vi "Get PK Info.vi"(8 "error in (no error)":errorcluster, 11 "FK Ring in":refnum<class "FK Ring.lvclass">) -> (0 "error out":errorcluster, 3 "FK Ring out":refnum<class "FK Ring.lvclass">)   [LabVIEW 2020, in "FK Ring.lvclass"]
uses:
  FK Ring.lvclass
  C:/Users/User/Desktop/Raman Program/Database OOP/source/Field/Field.lvclass
  Field/Field.lvclass/Field.ctl
  FK Ring.lvclass/FK Ring.ctl
  Database/Database.lvclass
  Field/Field.lvclass
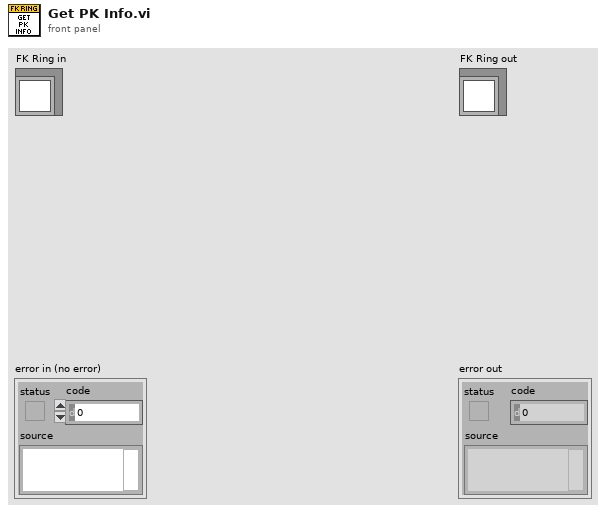
[diagram p1: front panel]
types:
  T1 = typedef "foreign key properties.ctl" = cluster{"FK Table":string, "FK Column":string, "PK Table":string, "PK Column":string, "PK Display Column":string}
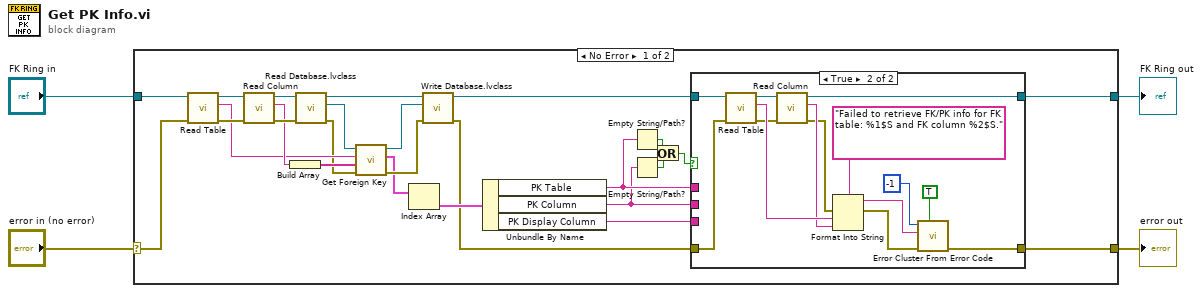
[diagram p0: block diagram]
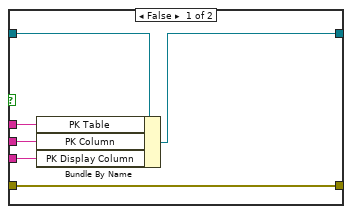
[diagram p2: hidden frame]
diagram:
  n1 = case shown="No Error" "error in (no error)" {
    selector: "error in (no error)" -> [w26 w52]
    tunnel: [w7 w52] -> w3
    tunnel: [w5 w51] -> w1
    tunnel: "FK Ring in" -> [w30 w51]
    frame No Error {
      n2 = call "Read Table.vi"("error in (no error)"=w26, "Field in"=w30) -> ("error out"=w25:errorcluster, "Table"=w22:string, "Field out"=w29:refnum<class "FK Ring.lvclass">)  [unwired: 7 in]
      n3 = call "Read Column.vi"("error in (no error)"=w25, "Field in"=w29) -> ("error out"=w24:errorcluster, "Column"=w23:string, "Field out"=w28:refnum<class "FK Ring.lvclass">)  [unwired: 7 in]
      n4 = Build Array(w23) -> (w21:string[])
      n5 = call "Read Database.lvclass.vi"("error in (no error)"=w24, "Field in"=w28) -> ("error out"=w18:errorcluster, "Database.lvclass"=w20:refnum<class "Database.lvclass">, "Field out"=w27:refnum<class "FK Ring.lvclass">)  [unwired: 7 in]
      n6 = call-dynamic "Get Foreign Key.vi"("error in (no error)"=w18, "Column Name Array"=w21, "Table Name"=w22, "Database in"=w20) -> ("error out"=w17:errorcluster, "FK Properties Array"=w16:T1[], "Database out"=w19:refnum<class "Database.lvclass">)  [unwired: 5 in]
      n7 = Index Array(array=w16) -> (element=w15:T1)  [unwired: 1 in]
      n8 = call "Write Database.lvclass.vi"("error in (no error)"=w17, "Database.lvclass"=w19, "Field in"=w27) -> ("error out"=w13:errorcluster, "Field out"=w6:refnum<class "FK Ring.lvclass">)  [unwired: 7 in]
      n9 = Unbundle By Name(w15) -> ("PK Table"=w12:string, "PK Column"=w8:string, "PK Display Column"=w14:string)
      n10 = Empty String/Path?(string/path=w12) -> (empty?=w11:bool)
      n11 = Empty String/Path?(string/path=w8) -> (empty?=w10:bool)
      n12 = Or(x=w11, y=w10) -> (x .or. y?=w9:bool)
      n13 = case shown="True" w9 {
        tunnel: w12 -> [w36 _]
        tunnel: w8 -> [w35 _]
        tunnel: w14 -> [w34 _]
        tunnel: w13 -> [w33 w44]
        tunnel: [w33 w37] -> w7
        tunnel: w6 -> [w32 w46]
        tunnel: [w31 w45] -> w5
        frame False {
          n14 = Bundle By Name(cluster=w32, "PK Table"=w36, "PK Column"=w35, "PK Display Column"=w34) -> (w31:refnum<class "FK Ring.lvclass">)
        }
        frame True {
          n15 = call "Read Table.vi"("error in (no error)"=w44, "Field in"=w46) -> ("error out"=w43:errorcluster, "Table"=w48:string, "Field out"=w49:refnum<class "FK Ring.lvclass">)  [unwired: 7 in]
          n16 = call "Read Column.vi"("error in (no error)"=w43, "Field in"=w49) -> ("error out"=w42:errorcluster, "Column"=w47:string, "Field out"=w45:refnum<class "FK Ring.lvclass">)  [unwired: 7 in]
          n17 = Format Into String(format string="Failed to retrieve FK/PK info for FK table: %1$S and FK column %2$S.", error in=w42, w48, w47) -> (resulting string=w41:string, error out=w40:errorcluster)  [unwired: 1 in]
          n18 = call <vilib>:"Error Cluster From Error Code.vi"("show call chain? (False)"=TRUE, "error in (no error)"=w40, "error message (\"\")"=w41, "error code (0)"=-1) -> ("error out"=w37:errorcluster)  [unwired: 5 in]
        }
      }
    }
    frame Error {
    }
  }
  "error out" <- w3
  "FK Ring out" <- w1
